vi "Manual Label Print.vi"(8 "error in (no error)":errorcluster) -> (0 "error out":errorcluster)   [LabVIEW 2017]
panel:
  out "FINAL BARCODE":string
  in  "NO OF PRINT":u16=1 min=1 max=100 step=1
  in  "stop":bool
  in  "Print":bool
  out "VARIENT":string
  out "USER":string
  # "MANUAL LABEL PRINT"
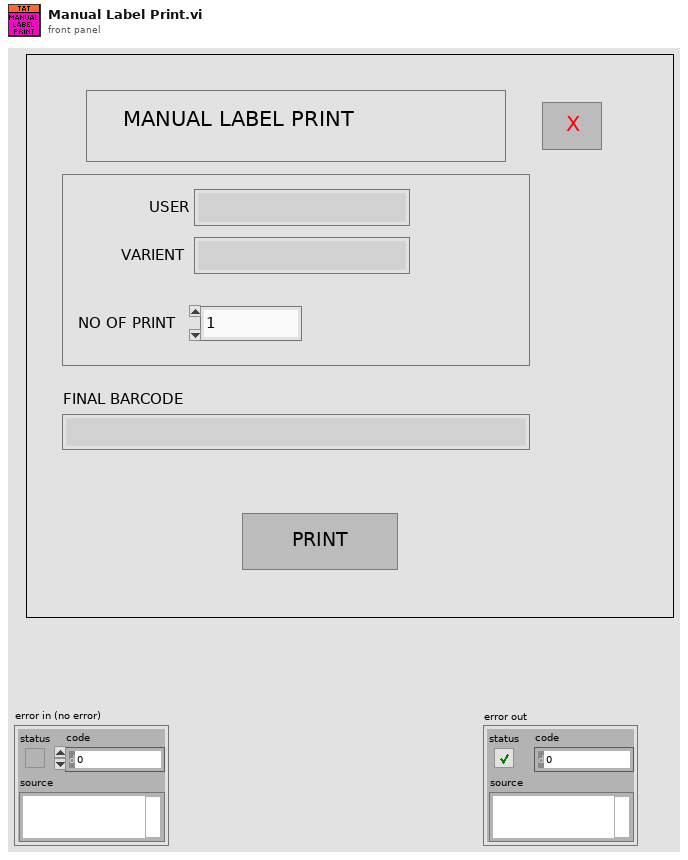
[diagram p1: front panel]
types:
  T1 = typedef "Recipe.ctl" = cluster{"Ass. Sensor Select":cluster{"Ass. Sensor Select":bool, "Camera-1 \nProg No.":u16, "Camera-2 \nProg No.":u16, "Gun \nProg No.":u16}, "Torque Sensor Select":cluster{"Torque Sensor-1":bool, "Torque Sensor-2":bool, "Torque Sensor-3":bool, "Torque Sensor-4":bool, "Torque Sensor-5":bool, "Torque Sensor-6":bool, "Torque Sensor-7":bool, "Torque Sensor-8":bool, "Torque Sensor-9":bool, "Torque Sensor-10":bool, "Torque Sensor-11":bool, "Torque Sensor-12":bool}, "Bin Seq. Select":cluster{"First Bin":u16, "Second Bin":u16, "Third Bin":u16, "Fourth Bin":u16, "Fifth Bin":u16, "Sixth Bin":u16, "Seventh Bin":u16, "Eighth Bin":u16, "Camera-1 Trig":u16, "Camera-2 Trig":u16}, "T-Bin Seq. Select":cluster{"First":u16, "Second":u16, "Third":u16, "Fourth":u16, "Fifth":u16, "Sixth":u16}, "Reference Barcode":cluster{"Spring Barcode":string, "Body Barcode":string, "14 Char of Barcode":string, "Final Barcode Length":string}, "Label Data":cluster{"Cust. Part No.":string, "TML Part No.":string, "Vendor Code":string, "Revision Level":string, "Part Description":string, "Vendor Name":string}}
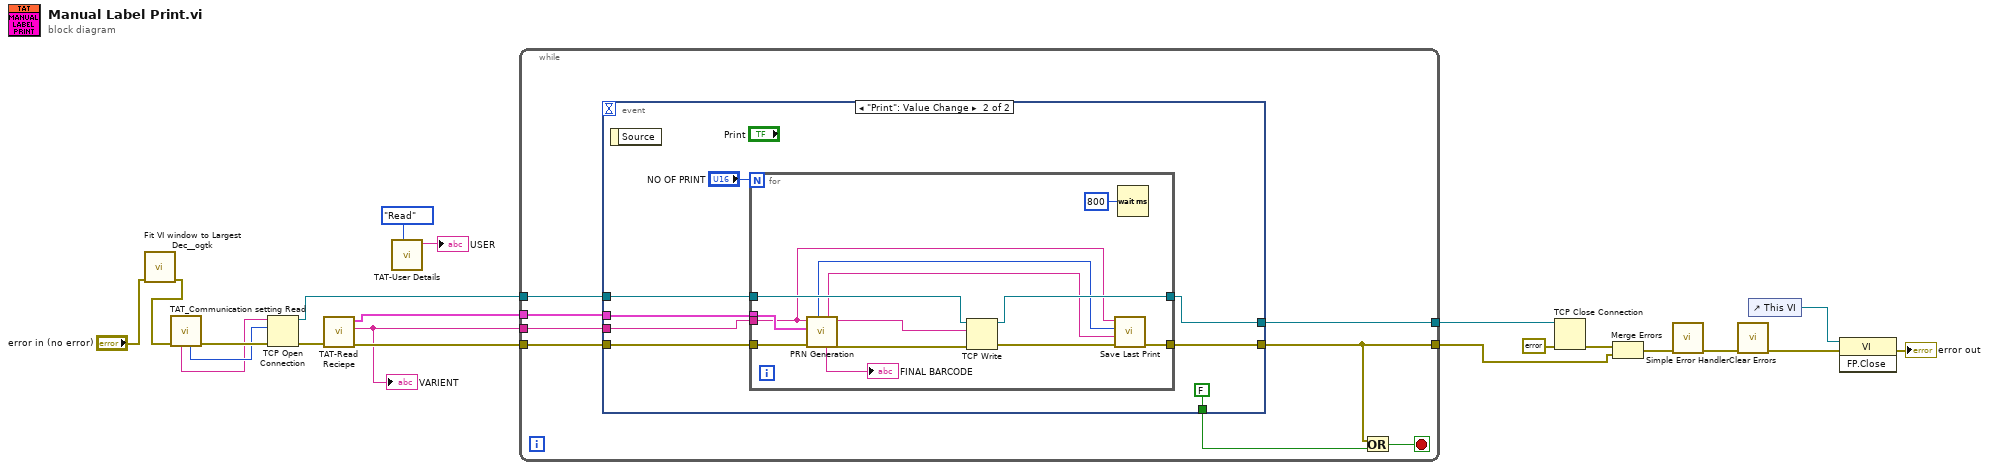
[diagram p0: block diagram]
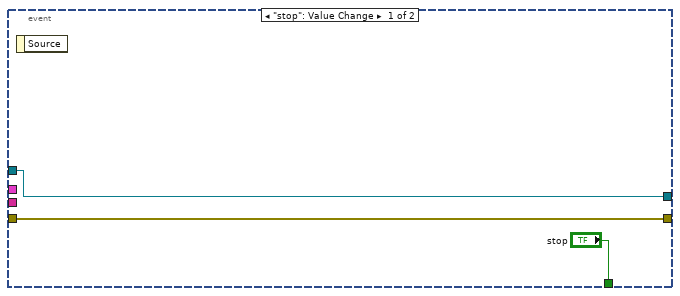
[diagram p2: hidden frame]
diagram:
  n1 = call <userlib>:"Fit VI window to Largest Dec__ogtk.vi"("error in (no error)"="error in (no error)") -> ("error out"=w1:errorcluster)  [unwired: 5 in, 1 out]
  n2 = call "TAT_Communication setting Read.vi"("error in (no error)"=w1) -> ("error out"=w5:errorcluster, "Printer Port"=w4:u32, "Printer IP"=w3:string)  [unwired: 3 in, 5 out]
  n3 = TCP Open Connection(address=w3, remote port or service name=w4, error in (no error)=w5) -> (connection ID=w18:refnum<k5>, error out=w6:errorcluster)  [unwired: 2 in]
  n4 = call "TAT-Read Reciepe.vi"("error in (no error)"=w6) -> ("error out"=w20:errorcluster, "Part Name"=w17:string, "Data To Load"=w19:T1)  [unwired: 8 in]
  "VARIENT" <- w17
  n5 = call "TAT-User Details.vi"("Enum"=enum16{"Read", "Write"}."Read") -> ("User Name Out"=→"USER":string)  [unwired: 9 in, 1 out]
  n6 = while {
    tunnel: w20 -> [w26]
    tunnel: w19 -> [w28]
    tunnel: w18 -> [w27]
    tunnel: w17 -> [w25]
    tunnel: [w23] -> w13
    tunnel: [w22] -> w7
    stop <- w24 stop-if-true
    n7 = event shown="[1] \"Print\": Value Change" {
      selector: _ -> [_ _]
      dyn-events: _ -> [_ _]
      timeout: _ -> [_ _]
      tunnel: ["stop" FALSE ("stop")] -> w29
      tunnel: w28 -> [_ w38]
      tunnel: w27 -> [w30 w37]
      tunnel: w26 -> [w31 w39]
      tunnel: w25 -> [_ w34]
      tunnel: [w31 w35] -> w23
      tunnel: [w30 w36] -> w22
      event "stop": Value Change {
        n8 = event-data() -> ()  [unwired: 1 in, 1 out]
      }
      event "Print": Value Change {
        n9 = event-data() -> ()  [unwired: 1 in, 1 out]
        n10 = for {
          N: "NO OF PRINT" -> [_]
          tunnel: w38 -> [w52]
          tunnel: w34 -> [w44]
          tunnel: w37 -> [w49]
          tunnel: [w47] -> w36
          tunnel: w39 -> [w53]
          tunnel: [w45] -> w35
          n11 = call "PRN Generation.vi"("error in (no error)"=w53, "Ref Data"=w52, "File Name"=w44) -> ("error out"=w50:errorcluster, "PRN to Print"=w48:string, "Barcode"=→"FINAL BARCODE":string, "Printing Date"=w42:string, "SN"=w43:u32)  [unwired: 3 in, 1 out]
          n12 = TCP Write(connection ID=w49, data in=w48, error in (no error)=w50) -> (connection ID out=w47:refnum<k5>, error out=w46:errorcluster)  [unwired: 1 in, 1 out]
          n13 = call "Save Last Print.vi"("error in (no error)"=w46, "Printing Date"=w42, "SN"=w43, "Part Name"=w44) -> ("error out"=w45:errorcluster)  [unwired: 7 in]
          n14 = Wait (ms)(milliseconds to wait=u32 800) -> ()  [unwired: 1 out]
        }
      }
    }
    n15 = Or(x=w23, y=w29) -> (x .or. y?=w24:bool)
  }
  n16 = TCP Close Connection(connection ID=w7, error in (no error)=errorcluster {"status"=FALSE, "code"=0, "source"=""}) -> (error out=w14:errorcluster)  [unwired: 1 in, 1 out]
  n17 = Merge Errors(w14, w13) -> (w12:errorcluster)
  n18 = call <vilib>:"Simple Error Handler.vi"("error in (no error)"=w12) -> ("error out"=w11:errorcluster)  [unwired: 4 in, 4 out]
  n19 = call <vilib>:"Clear Errors.vi"("error in (no error)"=w11) -> ("error out"=w10:errorcluster)  [unwired: 5 in, 1 out]
  n20 = control-ref of="This VI"() -> (w9:refnum<vi>)
  n21 = invoke class="VI" method="FP.Close"(reference=w9, error in=w10) -> (error out=→"error out":errorcluster)  [unwired: 1 in, 2 out]
